vi "Hook_03.vi"(7 "Mode":T1(ring), 8 "error in (no error)":errorcluster, 9 "data in":string, 10 "Port":u16=6342, 11 "Machine":string="localhost") -> (0 "error out":errorcluster, 3 "data out":string)   [LabVIEW 2011]
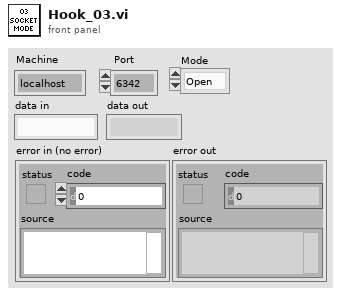
[diagram p1: front panel]
types:
  T1 = enum16{"Open", "R", "W", "R->W", "W->R", "Close"}
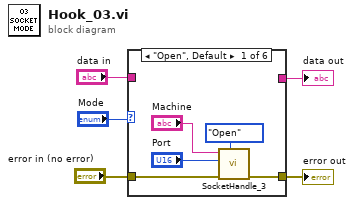
[diagram p0: block diagram]
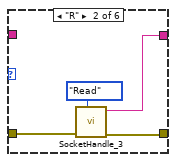
[diagram p2: hidden frame]
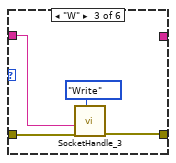
[diagram p3: hidden frame]
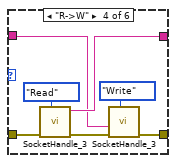
[diagram p4: hidden frame]
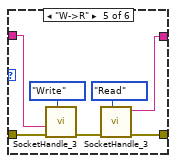
[diagram p5: hidden frame]
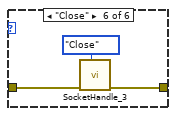
[diagram p6: hidden frame]
diagram:
  n1 = case shown="\"Open\", Default" "Mode" {
    tunnel: "error in (no error)" -> [w9 w13 w17 w23 w29 w34]
    tunnel: [w8 w12 w16 w21 w28 w33] -> w3
    tunnel: [_ w11 _ w20 w26 _] -> w2
    tunnel: "data in" -> [_ _ w15 w19 w27 _]
    frame "Open", Default {
      n2 = call "SocketHandle_3.vi"("Mode"=enum16{"Open", "Read", "Write", "Close"}."Open", "error in (no error)"=w9, "Port"="Port", "Machine"="Machine") -> ("error out"=w8:errorcluster)  [unwired: 6 in, 1 out]
    }
    frame "R" {
      n3 = call "SocketHandle_3.vi"("Mode"=enum16{"Open", "Read", "Write", "Close"}."Read", "error in (no error)"=w13) -> ("error out"=w12:errorcluster, "data out"=w11:string)  [unwired: 8 in]
    }
    frame "W" {
      n4 = call "SocketHandle_3.vi"("Mode"=enum16{"Open", "Read", "Write", "Close"}."Write", "error in (no error)"=w17, "data in"=w15) -> ("error out"=w16:errorcluster)  [unwired: 7 in, 1 out]
    }
    frame "R->W" {
      n5 = call "SocketHandle_3.vi"("Mode"=enum16{"Open", "Read", "Write", "Close"}."Read", "error in (no error)"=w23) -> ("error out"=w22:errorcluster, "data out"=w20:string)  [unwired: 8 in]
      n6 = call "SocketHandle_3.vi"("Mode"=enum16{"Open", "Read", "Write", "Close"}."Write", "error in (no error)"=w22, "data in"=w19) -> ("error out"=w21:errorcluster)  [unwired: 7 in, 1 out]
    }
    frame "W->R" {
      n7 = call "SocketHandle_3.vi"("Mode"=enum16{"Open", "Read", "Write", "Close"}."Write", "error in (no error)"=w29, "data in"=w27) -> ("error out"=w30:errorcluster)  [unwired: 7 in, 1 out]
      n8 = call "SocketHandle_3.vi"("Mode"=enum16{"Open", "Read", "Write", "Close"}."Read", "error in (no error)"=w30) -> ("error out"=w28:errorcluster, "data out"=w26:string)  [unwired: 8 in]
    }
    frame "Close" {
      n9 = call "SocketHandle_3.vi"("Mode"=enum16{"Open", "Read", "Write", "Close"}."Close", "error in (no error)"=w34) -> ("error out"=w33:errorcluster)  [unwired: 8 in, 1 out]
    }
  }
  "error out" <- w3
  "data out" <- w2
